vi "Replace Resource.vi"(6 "binary data":string, 8 "error in (no error)":errorcluster, 9 "Type":string, 10 "Palette Type":T1=-1 items=["Functions"=-1, "Controls"=-2], 11 "resources in":T2 {"type" format="%.0x"}) -> (0 "error out":errorcluster, 2 "Palette Type":T1=-1 items=["Functions"=-1, "Controls"=-2], 3 "resources out":T2 {"type" format="%.0x"})   [LabVIEW 2020, in "Palette Menu.lvlib" / "ResMgr.lvlib"]
uses:
  <vilib>/Palette API/ResMgr/ResMgr.lvlib
  <vilib>/Palette API/Palette Menu/Private Type Define/Resources.ctl
  <vilib>/Palette API/Palette Menu/Public Type Define/Palette type.ctl
  <vilib>/Palette API/ResMgr/Resource.ctl
  <vilib>/Palette API/Palette Menu/Palette Menu.lvlib
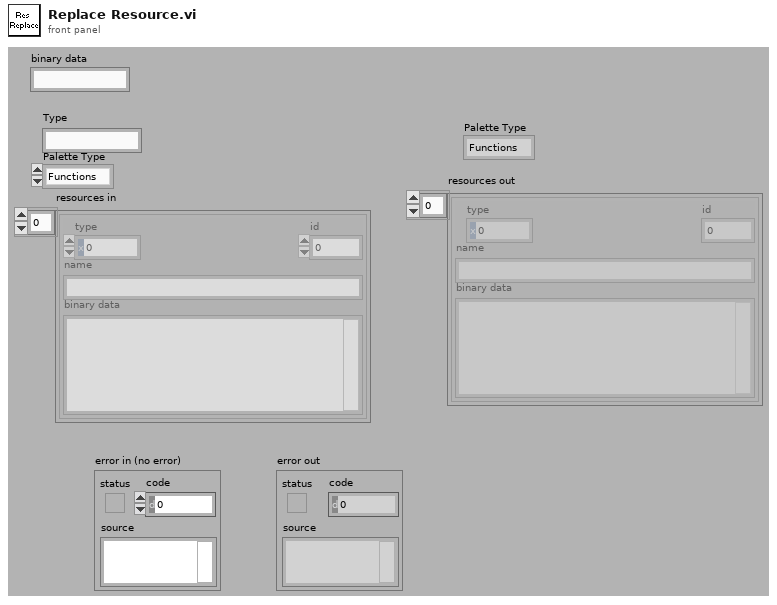
[diagram p1: front panel]
types:
  T1 = typedef "Palette Menu.lvlib/Palette type.ctl" = i32
  T2 = typedef "Palette Menu.lvlib/Resources.ctl" = cluster{"type":u32, "id":i32, "name":string, "binary data":string}[]
  T3 = typedef "Palette Menu.lvlib/ResMgr.lvlib/Resource.ctl" = cluster{"type":u32, "id":i32, "name":string, "binary data":string}
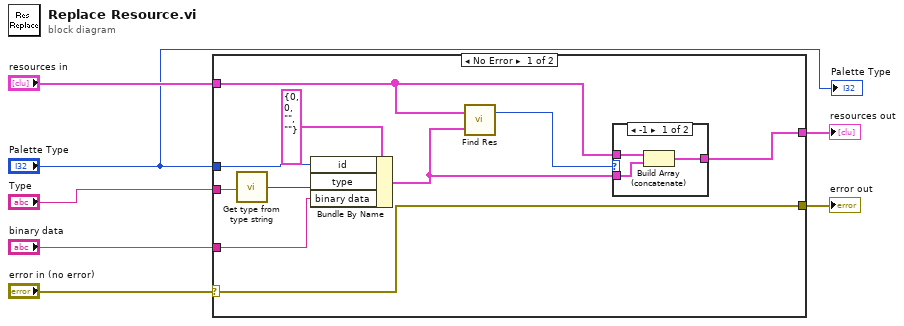
[diagram p0: block diagram]
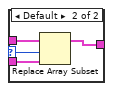
[diagram p2: hidden frame]
diagram:
  n1 = case shown="No Error" "error in (no error)" {
    selector: "error in (no error)" -> [w16 w26]
    tunnel: [w16 w26] -> w6
    tunnel: "resources in" -> [w17 w25]
    tunnel: [w8 w25] -> w4
    tunnel: "Palette Type" -> [w13 _]
    tunnel: "Type" -> [w12 _]
    tunnel: "binary data" -> [w11 _]
    frame No Error {
      n2 = call <vilib>:"Get type from type string.vi"("type string"=w12) -> ("type"=w15:u32)
      n3 = Bundle By Name(cluster=T3 {"type"=0, "id"=0, "name"="", "binary data"=""} ("resource info 2"), "id"=w13, "type"=w15, "binary data"=w11) -> (w9:T3)
      n4 = call <vilib>:"Find Res.vi"("info to match"=w9, "resources"=w17) -> ("index"=w10:i32)  [unwired: 1 out]
      n5 = case shown="-1" w10 {
        selector: w10 -> [_ w21]
        tunnel: [w18 w24] -> w8
        tunnel: w17 -> [w20 w23]
        tunnel: w9 -> [w19 w22]
        frame -1 {
          n6 = Build Array (concatenate)(w20, w19) -> (w18:T3[])
        }
        frame Default {
          n7 = Replace Array Subset(array=w23, new element=w22, index=w21) -> (w24:T2)
        }
      }
    }
    frame Error {
    }
  }
  "error out" <- w6
  "resources out" <- w4
  "Palette Type" <- "Palette Type"
